vi "Broadcast Diagnostic.vi"(8 "error in (no error)":errorcluster, 11 "interface object in":refnum<k20>) -> (0 "error out":errorcluster, 3 "interface object out":refnum<k20>)   [LabVIEW 2014]
uses:
  <vilib>/RioEmbeddedCAN/RioEmbeddedCAN.llb/CANWait.vi
  <vilib>/RioEmbeddedCAN/RioEmbeddedCAN.llb/CANWaitTransmitComplete.vi
  <vilib>/RioEmbeddedCAN/RioEmbeddedCAN.llb/CANWrite.vi
panel:
  in  "CAN Offset":u32=512 format="%x"
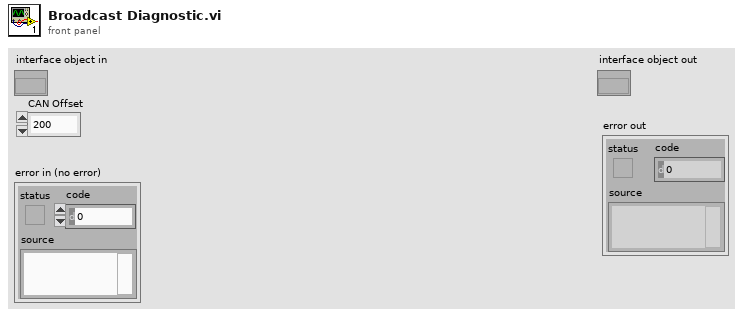
[diagram p1: front panel]
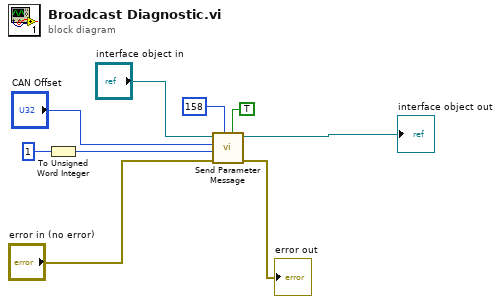
[diagram p0: block diagram]
diagram:
  n1 = To Unsigned Word Integer(number=u16 1) -> (unsigned 16bit integer=w2:u16)
  n2 = call "Send Parameter Message.vi"("Write?"=TRUE, "Param Address"=i16 158, "error in (no error)"="error in (no error)", "Data"=w2, "CAN Offset"="CAN Offset", "interface object in"="interface object in") -> ("error out"=→"error out":errorcluster, "interface object out"=→"interface object out":refnum<k20>)  [unwired: 4 in]
